vi "acqWaveform2chn.vi"(4 "error in (no error)":errorcluster, 5 "Channel":i8=1, 6 "Points":u32=5000 max=7000, 7 "OSC in":refnum<visa-resource-name>) -> (0 "error out":errorcluster, 1 "Voltage sequence":dbl[](array[numeric]), 2 "time sequence":dbl[](array[numeric]), 3 "OSC out":refnum<visa-resource-name>)   [LabVIEW 2016]
panel:
  out "XY Graph":cluster{dbl[], dbl[]}(graph)
  out "String":string
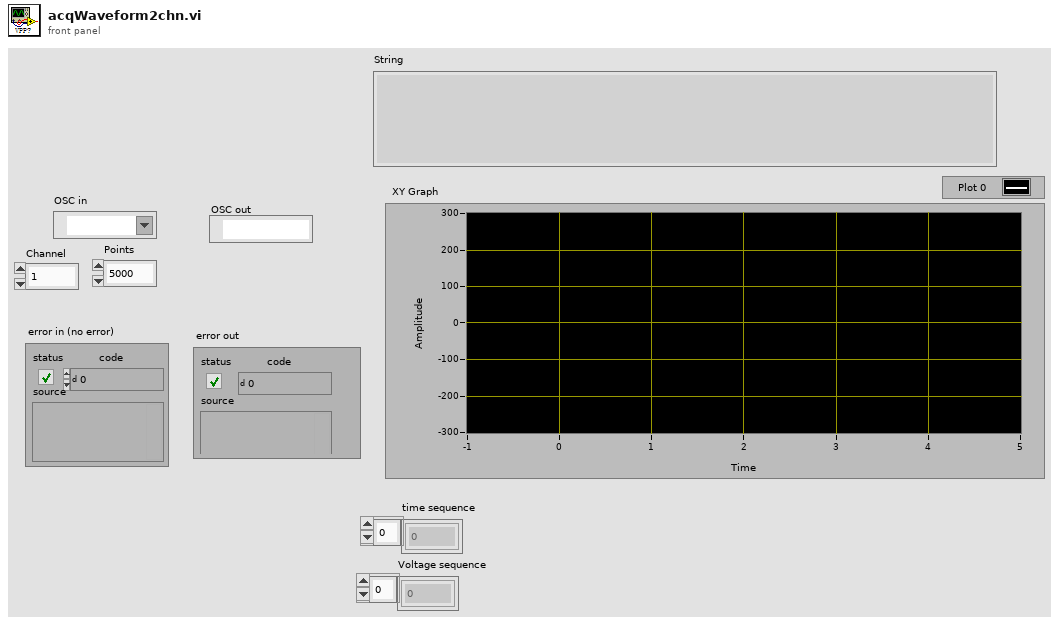
[diagram p1: front panel]
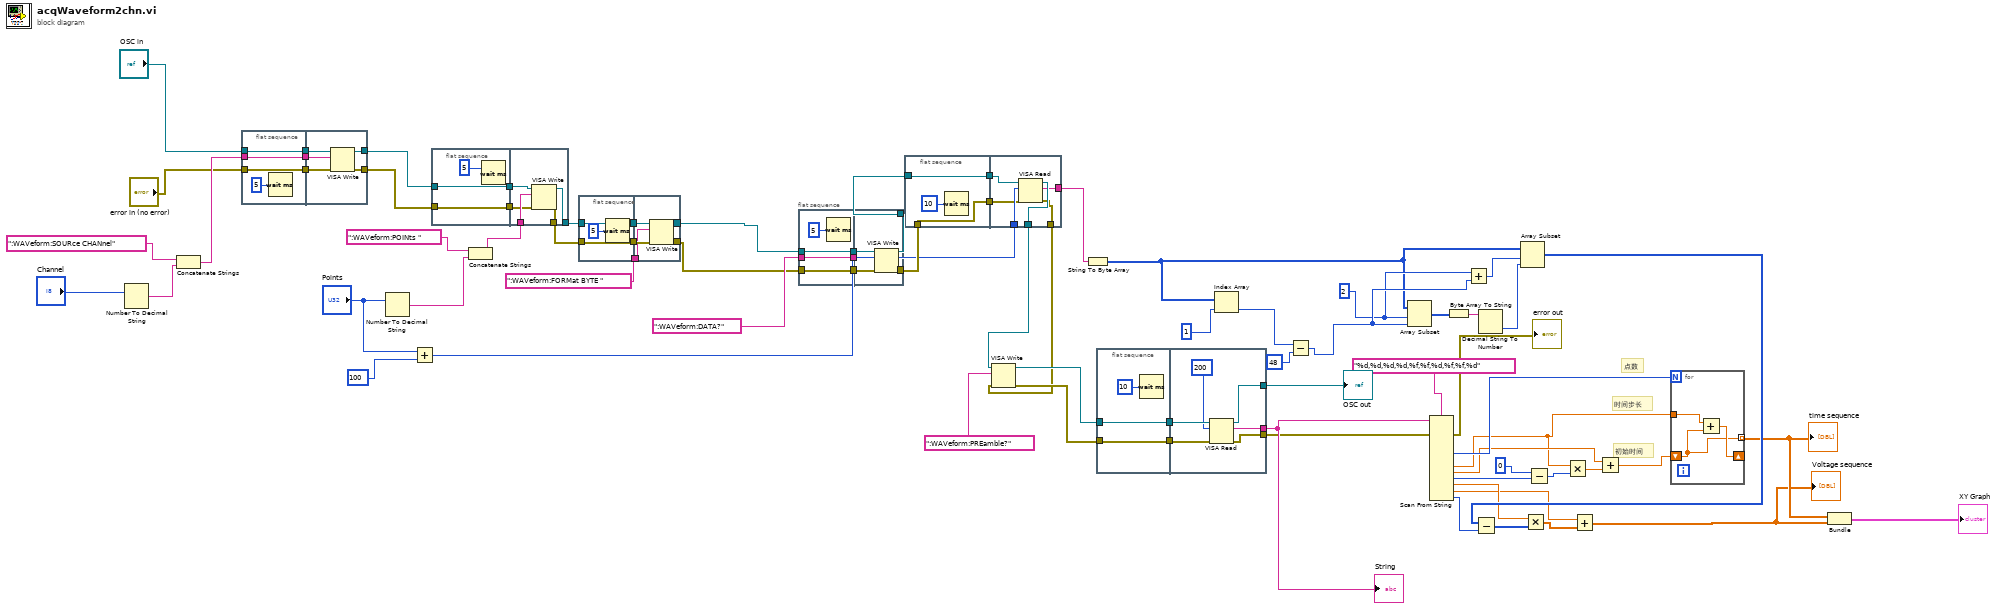
[diagram p0: block diagram]
diagram:
  w52 = 2
  # "初始时间"
  # "时间步长"
  # "点数"
  n1 = Number To Decimal String(number="Channel") -> (decimal integer string=w72:string)  [unwired: 1 in]
  n2 = Concatenate Strings(":WAVeform:SOURce CHANnel", w72) -> (w71:string)
  n3 = flat-sequence {
    tunnel: "error in (no error)" -> [w76]
    tunnel: "OSC in" -> [w77]
    tunnel: w71 -> [w78]
    tunnel: [w78] -> w14
    tunnel: [w77] -> w13
    tunnel: [w76] -> w12
    tunnel: [w82] -> w67
    tunnel: [w81] -> w66
    tunnel: w14 -> [w83]
    tunnel: w13 -> [w80]
    tunnel: w12 -> [w79]
    frame #0 {
      n4 = Wait (ms)(milliseconds to wait=u32 5) -> ()  [unwired: 1 out]
    }
    frame #1 {
      n5 = VISA Write(VISA resource name=w80, write buffer=w83, error in (no error)=w79) -> (VISA resource name out=w81:refnum<visa-resource-name>, error out=w82:errorcluster)  [unwired: 1 out]
    }
  }
  n6 = Number To Decimal String(number="Points") -> (decimal integer string=w70:string)  [unwired: 1 in]
  n7 = Add(x="Points", y=100) -> (x+y=w19:u32)
  n8 = flat-sequence {
    tunnel: w66 -> [w85]
    tunnel: w67 -> [w86]
    tunnel: [w86] -> w11
    tunnel: [w85] -> w10
    tunnel: w68 -> [w91]
    tunnel: [w88] -> w65
    tunnel: [w87] -> w64
    tunnel: w11 -> [w90]
    tunnel: w10 -> [w89]
    frame #0 {
      n9 = Wait (ms)(milliseconds to wait=u32 5) -> ()  [unwired: 1 out]
    }
    frame #1 {
      n10 = VISA Write(VISA resource name=w89, write buffer=w91, error in (no error)=w90) -> (VISA resource name out=w88:refnum<visa-resource-name>, error out=w87:errorcluster)  [unwired: 1 out]
    }
  }
  n11 = Concatenate Strings(":WAVeform:POINts ", w70) -> (w68:string)
  n12 = flat-sequence {
    tunnel: w64 -> [w93]
    tunnel: w65 -> [w94]
    tunnel: [w94] -> w9
    tunnel: [w93] -> w8
    tunnel: ":WAVeform:FORMat BYTE " -> [w97]
    tunnel: w9 -> [w99]
    tunnel: w8 -> [w98]
    tunnel: [w96] -> w4
    tunnel: [w95] -> w3
    frame #0 {
      n13 = Wait (ms)(milliseconds to wait=u32 5) -> ()  [unwired: 1 out]
    }
    frame #1 {
      n14 = VISA Write(VISA resource name=w99, write buffer=w97, error in (no error)=w98) -> (VISA resource name out=w96:refnum<visa-resource-name>, error out=w95:errorcluster)  [unwired: 1 out]
    }
  }
  n15 = flat-sequence {
    tunnel: w3 -> [w101]
    tunnel: w4 -> [w102]
    tunnel: ":WAVeform:DATA?" -> [w103]
    tunnel: [w103] -> w7
    tunnel: [w102] -> w6
    tunnel: [w101] -> w5
    tunnel: [w105] -> w24
    tunnel: [w104] -> w22
    tunnel: w7 -> [w108]
    tunnel: w6 -> [w107]
    tunnel: w5 -> [w106]
    frame #0 {
      n16 = Wait (ms)(milliseconds to wait=u32 5) -> ()  [unwired: 1 out]
    }
    frame #1 {
      n17 = VISA Write(VISA resource name=w107, write buffer=w108, error in (no error)=w106) -> (VISA resource name out=w105:refnum<visa-resource-name>, error out=w104:errorcluster)  [unwired: 1 out]
    }
  }
  n18 = flat-sequence {
    tunnel: w24 -> [w110]
    tunnel: [w110] -> w23
    tunnel: w22 -> [w109]
    tunnel: [w109] -> w21
    tunnel: w23 -> [w112]
    tunnel: w21 -> [w113]
    tunnel: [w117] -> w2
    tunnel: [w116] -> w20
    tunnel: [w115] -> w1
    tunnel: w19 -> [w114]
    frame #0 {
      n19 = Wait (ms)(milliseconds to wait=u32 10) -> ()  [unwired: 1 out]
    }
    frame #1 {
      n20 = VISA Read(VISA resource name=w112, byte count=w114, error in (no error)=w113) -> (VISA resource name out=w117:refnum<visa-resource-name>, read buffer=w116:string, error out=w115:errorcluster)  [unwired: 1 out]
    }
  }
  n21 = VISA Write(VISA resource name=w2, write buffer=":WAVeform:PREamble?", error in (no error)=w1) -> (VISA resource name out=w48:refnum<visa-resource-name>, error out=w47:errorcluster)  [unwired: 1 out]
  n22 = String To Byte Array(string=w20) -> (unsigned byte array=w50:u8[])
  n23 = flat-sequence {
    tunnel: w47 -> [w119]
    tunnel: w48 -> [w120]
    tunnel: [w120] -> w18
    tunnel: [w119] -> w17
    tunnel: [w124] -> w46
    tunnel: [w122] -> w44
    tunnel: [w121] -> w43
    tunnel: w18 -> [w126]
    tunnel: w17 -> [w125]
    frame #0 {
      n24 = Wait (ms)(milliseconds to wait=u32 10) -> ()  [unwired: 1 out]
    }
    frame #1 {
      n25 = VISA Read(VISA resource name=w126, byte count=200, error in (no error)=w125) -> (VISA resource name out=w124:refnum<visa-resource-name>, read buffer=w122:string, error out=w121:errorcluster)  [unwired: 1 out]
    }
  }
  n26 = Index Array(array=w50, index=1) -> (element=w58:u8)
  n27 = Subtract(x=w58, y=48) -> (x-y=w53:i32)
  n28 = Array Subset(array=w50, index=w52, length=w53) -> (w56:u8[])
  n29 = Scan From String(format string="%d,%d,%d,%d,%f,%f,%d,%f,%f,%d", input string=w44, error in=w43) -> (error out=→"error out":errorcluster, output 3=w41:i32, output 5=w34:dbl, output 6=w36:dbl, output 7=w40:i32, output 8=w30:dbl, output 9=w29:dbl, output 10=w32:i32)  [unwired: 14 in, 2 out]
  n30 = Byte Array To String(unsigned byte array=w56) -> (string=w55:string)
  n31 = Add(x=w52, y=w53) -> (x+y=w51:i32)
  n32 = Decimal String To Number(string=w55) -> (number=w54:i32)  [unwired: 2 in, 1 out]
  n33 = Array Subset(array=w50, index=w51, length=w54) -> (w33:u8[])
  n34 = Subtract(x=w33, y=w32) -> (x-y=w31:i32[])
  n35 = Multiply(x=w30, y=w31) -> (x*y=w28:dbl[])
  n36 = Subtract(x=0, y=w40) -> (x-y=w38:i32)
  n37 = Multiply(x=w34, y=w38) -> (x*y=w37:dbl)
  n38 = Add(x=w29, y=w28) -> (x+y=w25:dbl[])
  "Voltage sequence" <- w25
  n39 = Add(x=w36, y=w37) -> (x+y=w35:dbl)
  n40 = for {
    N: w41 -> [_]
    shift-right: [w129] -> _
    shift-left: w35 -> [w127]
    tunnel: w34 -> [w128]
    tunnel: [w127] -> w27 mode=indexing
    n41 = Add(x=w128, y=w127) -> (x+y=w129:dbl)
  }
  "time sequence" <- w27
  n42 = Bundle(w27, w25) -> (→"XY Graph":cluster{dbl[], dbl[]})  [unwired: 1 in]
  "OSC out" <- w46
  "String" <- w44
